vi "Read Update Mode.vi"(9 "WaveformChart in":refnum<class "WaveformGraph.lvclass">) -> (3 "WaveformChart out":refnum<class "WaveformGraph.lvclass">, 4 "Update Mode":u8)   [LabVIEW 2014]
uses:
  WaveformGraph.lvclass
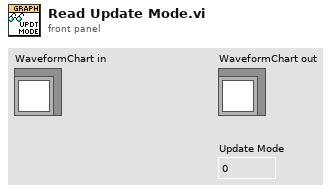
[diagram p1: front panel]
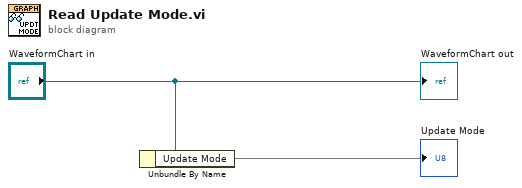
[diagram p0: block diagram]
diagram:
  n1 = Unbundle By Name("WaveformChart in") -> ("Update Mode"=→"Update Mode")
  "WaveformChart out" <- "WaveformChart in"
